vi "Initial Matrix.vi"   [LabVIEW 2014, in "NI_AALBase.lvlib"]
uses:
  NI_AALBase.lvlib
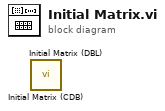
[diagram p0: block diagram]
diagram:
  n1 = call "Initial Matrix (CDB).vi"() -> ()  [unwired: 10 in, 2 out]
  n2 = call "Initial Matrix (DBL).vi"() -> ()  [unwired: 10 in, 2 out]
